vi "Test Harness.vi"() -> ()   [LabVIEW 2015, in "Command Handler.lvlib"]
uses:
  Command Handler.lvlib
  <vilib>/ActorFramework/Actor/Actor.lvclass
  Command Handler/Command Handler.lvclass
  <vilib>/ActorFramework/Stop Msg/Stop Msg.lvclass
  Command Handler Messages/Load Command Msg/Load Command Msg.lvclass
  Command Handler Messages/Execute Loaded Command Msg/Execute Loaded Command Msg.lvclass
  Command Handler Messages/Execute Command Msg/Execute Command Msg.lvclass
  Command Parent/Command.lvclass
  Command Handler Messages/Execute Loaded Commands Msg/Execute Loaded Commands Msg.lvclass
  Command Handler Messages/Return Events Msg/Return Events Msg.lvclass
panel:
  in  "Commands Folder":path
  out "Last Error Time":timestamp
  in  "Enable Command Handling":bool
  in  "Disable Command Handling":bool
  in  "Reload":bool
  out "Last Handler Error":errorcluster
  in  "Commands":string(combo)
  in  "Run Loaded Commands":bool
  in  "Front (T) Back (F)":bool
  in  "Run Next Loaded Command":bool
  in  "Execute Command":bool
  in  "Add Command":bool
  out "Completed Commands":string[](array[string])
  out "Commands Completed":i32
  out "Loaded Commands":string[](array[string])
  out "Commands Loaded":i32
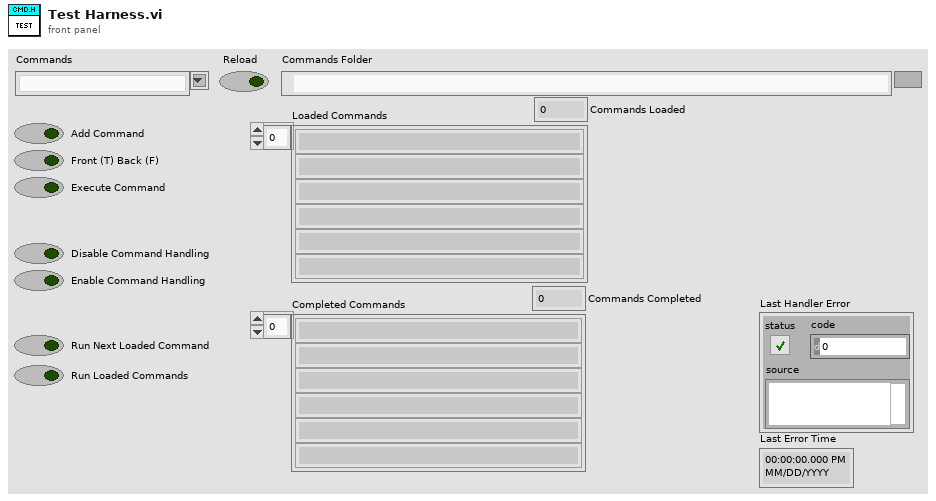
[diagram p1: front panel]
types:
  T1 = typedef "Command Handler.lvlib/Command Handler.lvclass/Event Cluster.ctl" = cluster{"Error Event":refnum<user-event>, "Command Done Event":refnum<user-event>, "Stopping Event":refnum<user-event>, "Data Update Event":refnum<user-event>}
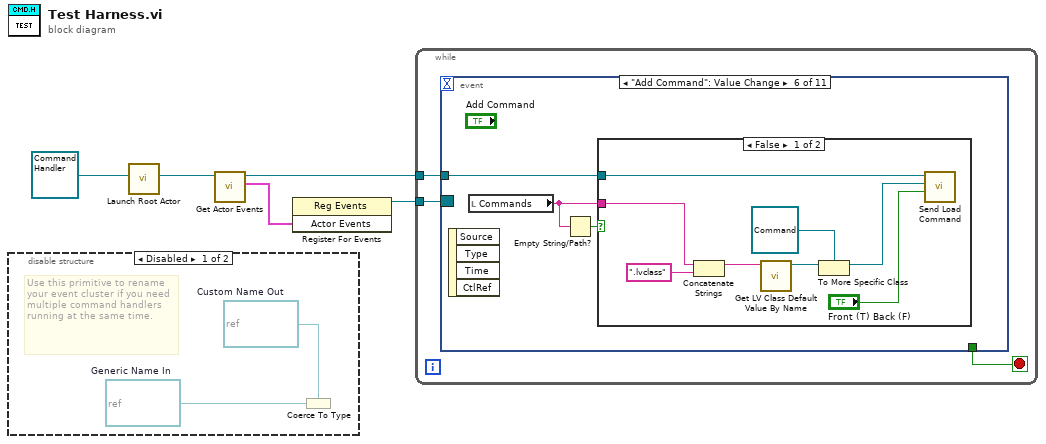
[diagram p0: block diagram]
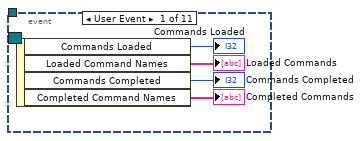
[diagram p3: hidden frame]
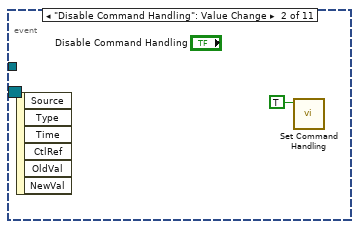
[diagram p4: hidden frame]
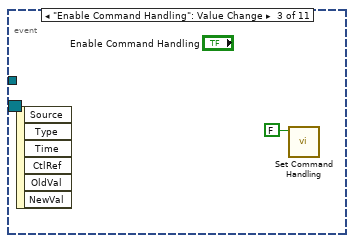
[diagram p5: hidden frame]
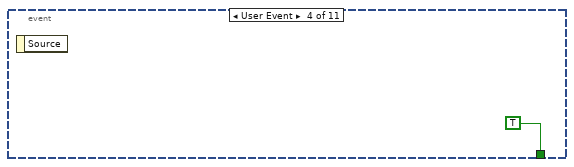
[diagram p6: hidden frame]
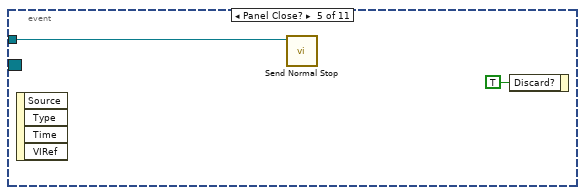
[diagram p7: hidden frame]
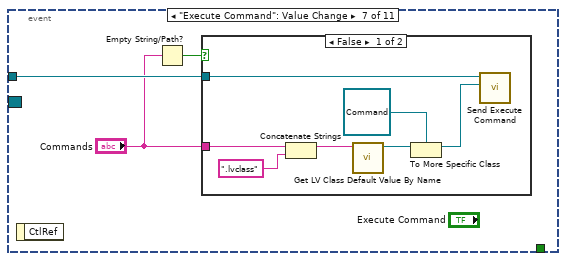
[diagram p9: hidden frame]
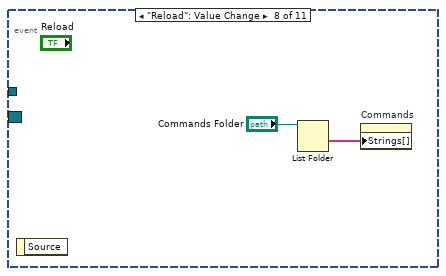
[diagram p11: hidden frame]
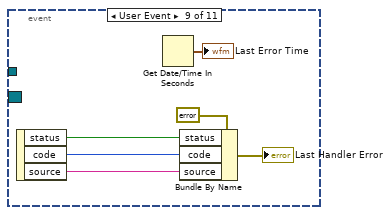
[diagram p12: hidden frame]
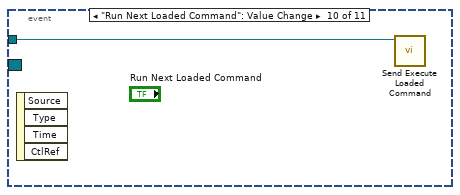
[diagram p13: hidden frame]
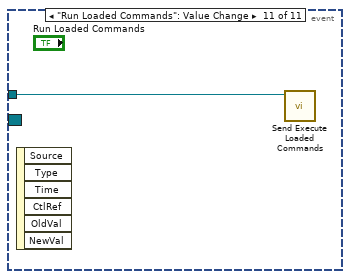
[diagram p14: hidden frame]
diagram:
  n1 = disable-structure shown="Disabled" {
    frame Disabled {
      w6 = refnum<user-event> refnum  # Custom Name Out
      w7 = refnum<user-event> refnum  # Generic Name In
      # "Use this primitive to rename your event cluster if you need multiple command handlers running at the same time."
      n2 = Coerce To Type(0:w7, 1:w6) -> ()  [unwired: 1 out]
    }
    frame Enabled {
    }
  }
  n3 = call <vilib>:"Launch Root Actor.vi"("Actor"=refnum<class "Command Handler.lvclass"> refnum ("Command Handler.lvlib:Command Handler.lvclass")) -> ("Actor's Enqueuer"=w1:refnum<class "Message Enqueuer.lvclass">)  [unwired: 9 in, 1 out]
  n4 = call "Get Actor Events.vi"("Message Enqueuer in"=w1) -> ("Actor Events"=w2:T1, "Message Enqueuer out"=w4:refnum<class "Message Enqueuer.lvclass">)  [unwired: 7 in, 2 out]
  n5 = register-events(w2) -> (reference out=w5:refnum<event-registration>)  [unwired: 2 in, 1 out]
  n6 = while {
    tunnel: w5 -> [w10]
    tunnel: w4 -> [w8]
    stop <- w9 stop-if-true
    n7 = event shown="[5] \"Add Command\": Value Change" {
      selector: w10 -> [_ _ _ _ _ _ _ _ _ _ _]
      dyn-events: _ -> [_ _ _ _ _ _ _ _ _ _ _]
      timeout: _ -> [_ _ _ _ _ _ _ _ _ _ _]
      tunnel: [_ _ _ TRUE _ _ _ _ _ _ _] -> w9
      tunnel: w8 -> [_ _ _ _ w19 w22 w33 _ _ w49 w50]
      event User Event {
        n8 = event-data() -> ("Commands Loaded"=→"Commands Loaded":i32, "Loaded Command Names"=→"Loaded Commands":string[], "Commands Completed"=→"Commands Completed":i32, "Completed Command Names"=→"Completed Commands":string[])  [unwired: 1 in]
      }
      event "Disable Command Handling": Value Change {
        n9 = event-data() -> ()  [unwired: 1 in, 6 out]
        n10 = call "Set Command Handling.vi"("Disable Command Handling"=TRUE ("Command Handling Stopped")) -> ()  [unwired: 10 in, 1 out]
      }
      event "Enable Command Handling": Value Change {
        n11 = event-data() -> ()  [unwired: 1 in, 6 out]
        n12 = call "Set Command Handling.vi"("Disable Command Handling"=FALSE ("Command Handling Stopped")) -> ()  [unwired: 10 in, 1 out]
      }
      event User Event {
        n13 = event-data() -> ()  [unwired: 1 in, 1 out]
      }
      event Panel Close? {
        n14 = event-data() -> ()  [unwired: 1 in, 4 out]
        n15 = call <vilib>:"Send Normal Stop.vi"("Message Enqueuer"=w19) -> ()  [unwired: 10 in, 1 out]
        n16 = event-data("Discard?"=TRUE) -> ()  [unwired: 1 in, 1 out]
      }
      event "Add Command": Value Change {
        n17 = event-data() -> ()  [unwired: 1 in, 4 out]
        n18 = local read "Commands"() -> (w21:string)
        n19 = Empty String/Path?(string/path=w21) -> (empty?=w20:bool)
        n20 = case shown="False" w20 {
          tunnel: w22 -> [w30 _]
          tunnel: w21 -> [w23 _]
          frame False {
            n21 = Concatenate Strings(w23, ".lvclass" ("string")) -> (w25:string)
            n22 = call <vilib>:"Get LV Class Default Value By Name.vi"("class name"=w25) -> ("object"=w28:refnum<class>)  [unwired: 9 in, 1 out]
            n23 = To More Specific Class(target class=refnum<class "Command.lvclass"> refnum ("Command.lvclass"), reference=w28) -> (specific class reference=w27:refnum<class "Command.lvclass">)  [unwired: 1 in, 1 out]
            n24 = call "Send Load Command.vi"("Front (T) Back (F)"="Front (T) Back (F)", "Command In"=w27, "Message Enqueuer"=w30) -> ()  [unwired: 7 in, 2 out]
          }
          frame True {
          }
        }
      }
      event "Execute Command": Value Change {
        n25 = event-data() -> ()  [unwired: 1 in, 1 out]
        n26 = Empty String/Path?(string/path="Commands") -> (empty?=w32:bool)
        n27 = case shown="False" w32 {
          tunnel: w33 -> [w40 _]
          tunnel: "Commands" -> [w34 _]
          frame False {
            n28 = Concatenate Strings(w34, ".lvclass" ("string")) -> (w37:string)
            n29 = call <vilib>:"Get LV Class Default Value By Name.vi"("class name"=w37) -> ("object"=w39:refnum<class>)  [unwired: 9 in, 1 out]
            n30 = To More Specific Class(target class=refnum<class "Command.lvclass"> refnum ("Command.lvclass"), reference=w39) -> (specific class reference=w36:refnum<class "Command.lvclass">)  [unwired: 1 in, 1 out]
            n31 = call "Send Execute Command.vi"("Command"=w36, "Message Enqueuer"=w40) -> ()  [unwired: 8 in, 2 out]
          }
          frame True {
          }
        }
      }
      event "Reload": Value Change {
        n32 = event-data() -> ()  [unwired: 1 in, 1 out]
        n33 = List Folder(path="Commands Folder") -> (folder names=w42:string[])  [unwired: 3 in, 3 out]
        n34 = property on="Commands" class="CmbBox"("Strings[]"=w42) -> ()  [unwired: 2 in, 2 out]
      }
      event User Event {
        n35 = event-data() -> ("status"=w47:bool, "code"=w46:i32, "source"=w45:string)  [unwired: 1 in]
        n36 = Get Date/Time In Seconds() -> (seconds since 1Jan1904=→"Last Error Time":timestamp)
        n37 = Bundle By Name(cluster=errorcluster {"status"=FALSE, "code"=0, "source"=""} ("error constant"), "status"=w47, "code"=w46, "source"=w45) -> (→"Last Handler Error":errorcluster)
      }
      event "Run Next Loaded Command": Value Change {
        n38 = event-data() -> ()  [unwired: 1 in, 4 out]
        n39 = call "Send Execute Loaded Command.vi"("Message Enqueuer"=w49) -> ()  [unwired: 9 in, 2 out]
      }
      event "Run Loaded Commands": Value Change {
        n40 = event-data() -> ()  [unwired: 1 in, 6 out]
        n41 = call "Send Execute Loaded Commands.vi"("Message Enqueuer"=w50) -> ()  [unwired: 9 in, 2 out]
      }
    }
  }
